vi "GlobalClimber.vi"() -> ()   [LabVIEW 2023]
panel:
  out "OUT_Climber 2":bool
  out "OUT_Climber":dbl
  out "REF_Climber":string
  # "DEVICE REFERENCE NAMES"
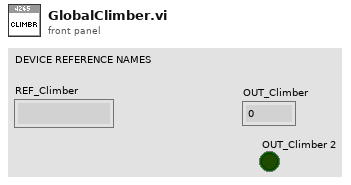
[diagram p1: front panel]
diagram:
